vi "StateMachine.vi"() -> ()   [LabVIEW 2025]
doc: "Implements a state machine using a string-based approach with states such as 'Start', 'Calculate', and 'Stop'. Each state executes specific logic based on its role.Start state defaults each input with 0. Calculate state calculates the addition of 2 numbers and stop state stops the execution."
panel:
  out "result":dbl
  in  "num 1":dbl
  in  "num 2":dbl
  in  "?":bool
  # "Implemented State machine with different states of a string like start, calculate, stop and based on state implemented the logic"
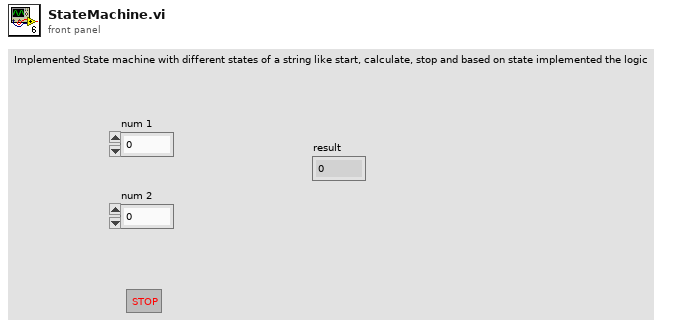
[diagram p1: front panel]
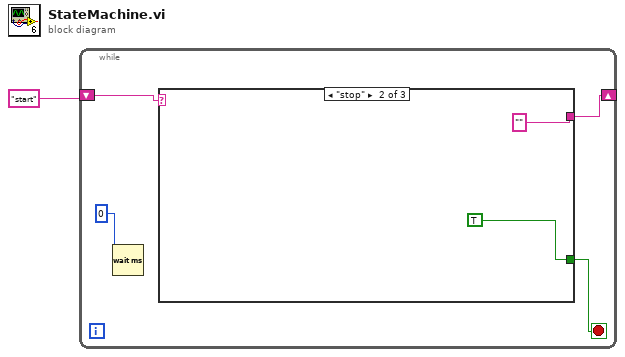
[diagram p0: block diagram]
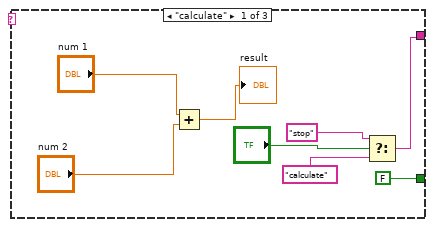
[diagram p2: hidden frame]
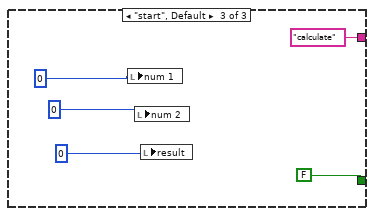
[diagram p3: hidden frame]
diagram:
  n1 = while {
    shift-right: [w4] -> _
    shift-left: "start" -> [w5]
    stop <- w3 stop-if-true
    n2 = Wait (ms)(milliseconds to wait=0) -> ()  [unwired: 1 out]
    n3 = case shown="\"stop\"" w5 {
      tunnel: [w6 "" "calculate"] -> w4
      tunnel: [FALSE TRUE FALSE] -> w3
      frame "calculate" {
        n4 = Add(x="num 1", y="num 2") -> (x+y=→"result":dbl)
        n5 = Select(t="stop", s="?", f="calculate") -> (s? t:f=w6:string)
      }
      frame "stop" {
      }
      frame "start", Default {
        n6 = local write "num 1"(0) -> ()
        n7 = local write "num 2"(0) -> ()
        n8 = local write "result"(0) -> ()
      }
    }
  }
